vi "Main_maszyna.vi"() -> ()   [LabVIEW 2013]
doc: "Use this template to build a standard state machine design pattern. Each state executes code and determines which state to transition to. Contrast this design pattern with the User Interface Event Handler pattern, in which code executes in response to user actions. Contrast this design pattern also with the Queued Message Handler pattern, in which each message handling code can queue zero or more new messages.\nNote: This template does not contain the most recent programming guidelines recommended by National Instruments. For a complete, project-based implementation of the Standard State Machine pattern, use the Create Project dialog box instead of this template."
uses:
  inne pliki/Stany.ctl
  inne pliki/Params.ctl
  inne pliki/Data.ctl
  inne pliki/Akcje czas FVG.ctl
  <vilib>/Utility/error.llb/DialogType.ctl
  <vilib>/Utility/file.llb/Write To Spreadsheet File (DBL).vi
panel:
  out "path out":path
  in  "Generuj (F)":bool
  in  "Error?":bool
  out "Czas do końca pomiaru":dbl
  in  "bStopPomiar":bool
  out "Warning text":string
  out "Warning":bool
  in  "Temp limits":T1={"Max (25)"=22.0, "Min (0)"=0.0}
  out "Waveform Chart":cluster{"Temperatura":dbl, "Średnia":dbl}(graph)
  in  "Akcje":T2
  out "Stan aktualny":T3
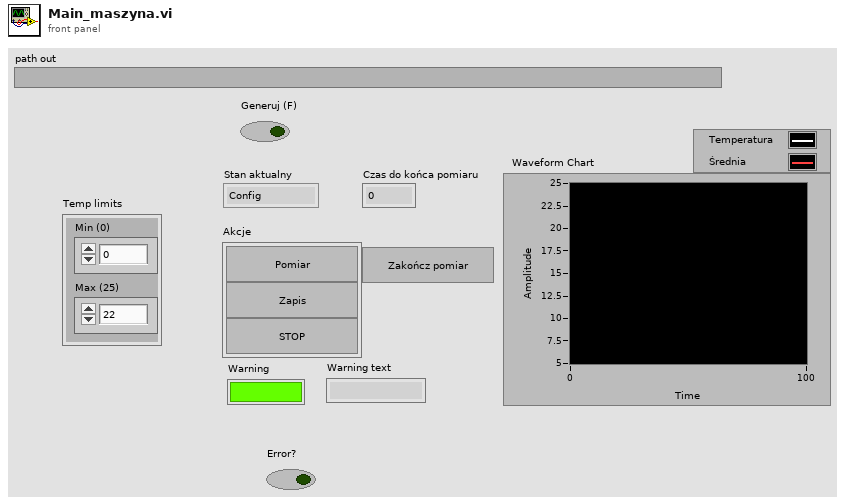
[diagram p1: front panel]
types:
  T1 = typedef "Params.ctl" = cluster{"Max (25)":dbl, "Min (0)":dbl}
  T2 = cluster{"bPomiar":bool, "bZapis":bool, "bSTOP":bool}
  T3 = typedef "Stany.ctl" = enum16{"Config", "IDLE", "Measure", "Analyze", "Display", "STOP", "Save", "Error", "Error end"}
  T4 = typedef "Data.ctl" = cluster{"Temperatura":dbl, "Średnia":dbl, "Warning":bool, "Warning text ":string, "Temp limits":T1, "Temp Array":dbl[], "Sternia Array":dbl[]}
  T5 = typedef "Akcje czas FVG.ctl" = enum16{"Reset", "Wait"}
  T6 = typedef "DialogType.ctl" = u16
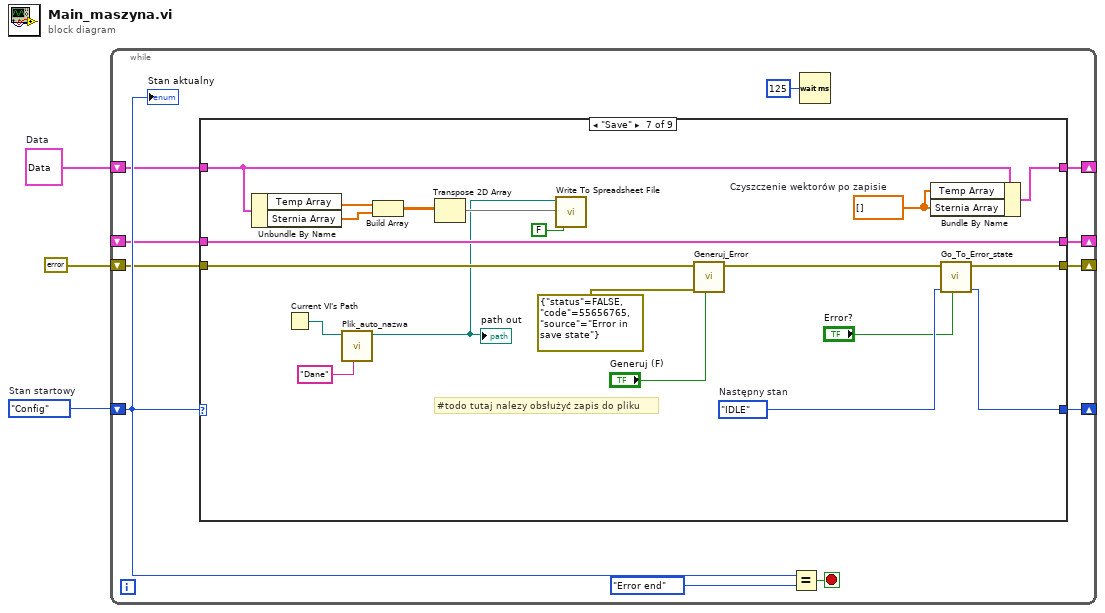
[diagram p0: block diagram]
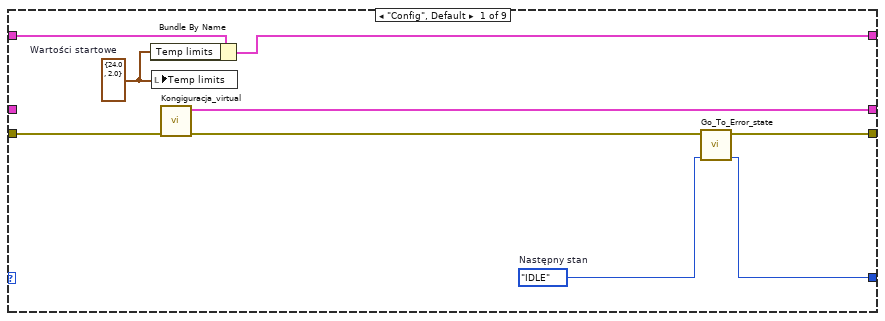
[diagram p2: hidden frame]
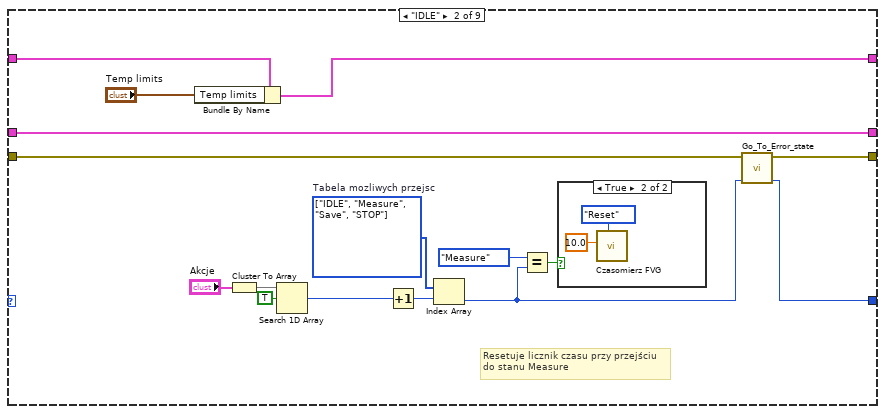
[diagram p3: hidden frame]
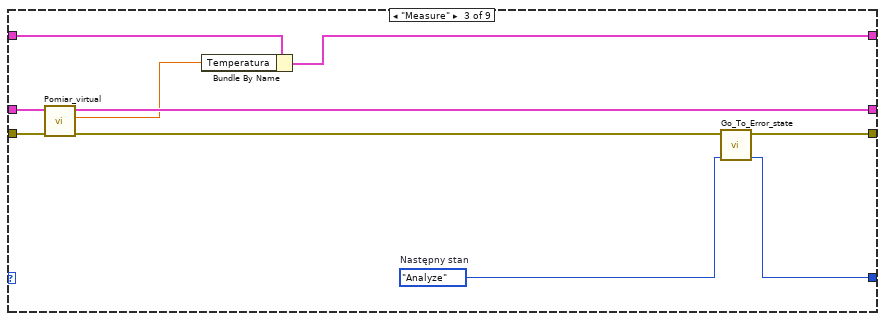
[diagram p5: hidden frame]
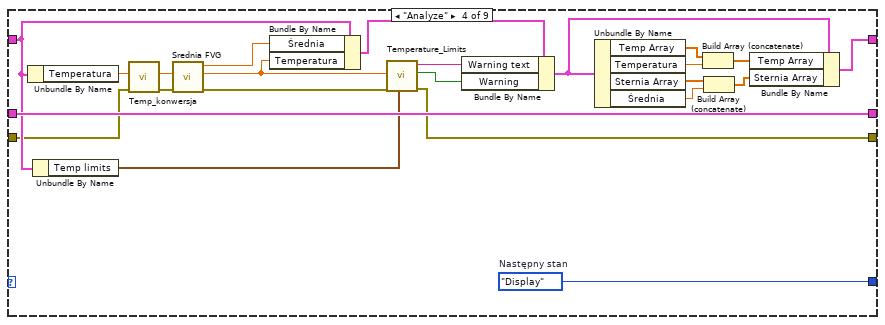
[diagram p6: hidden frame]
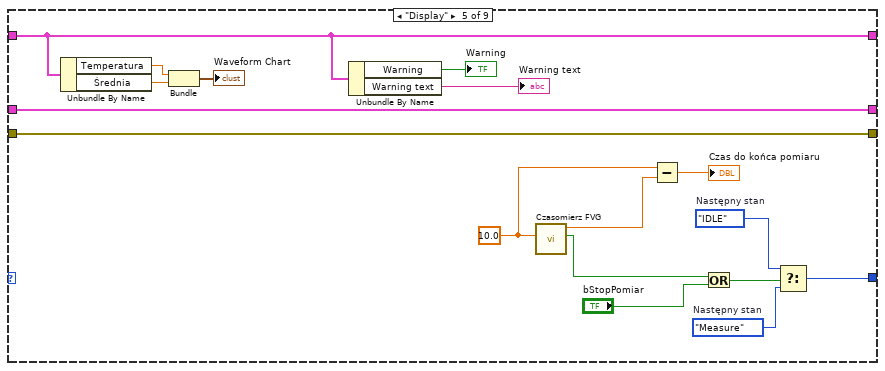
[diagram p7: hidden frame]
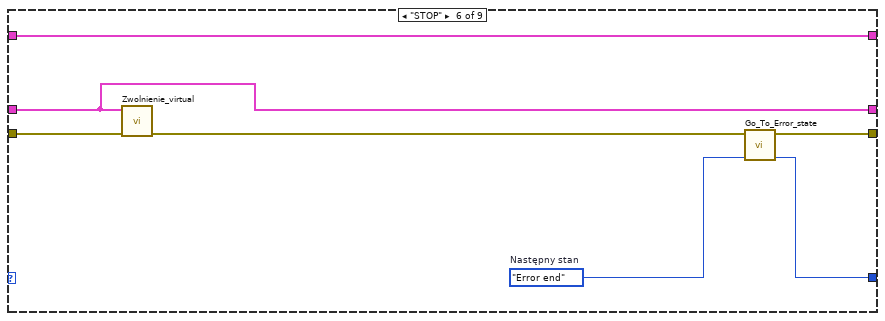
[diagram p8: hidden frame]
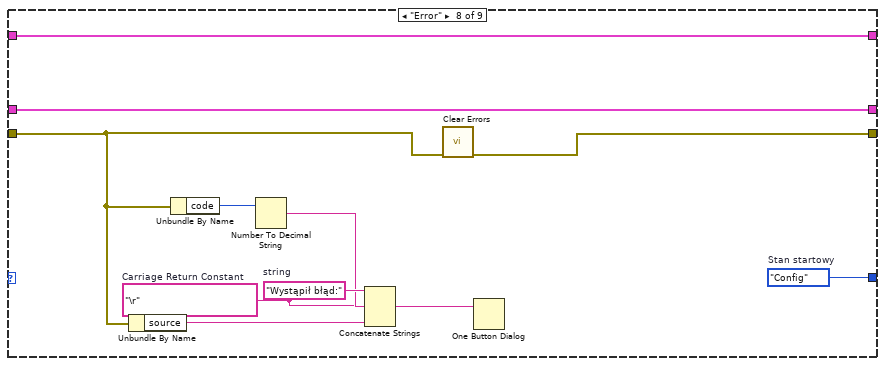
[diagram p9: hidden frame]
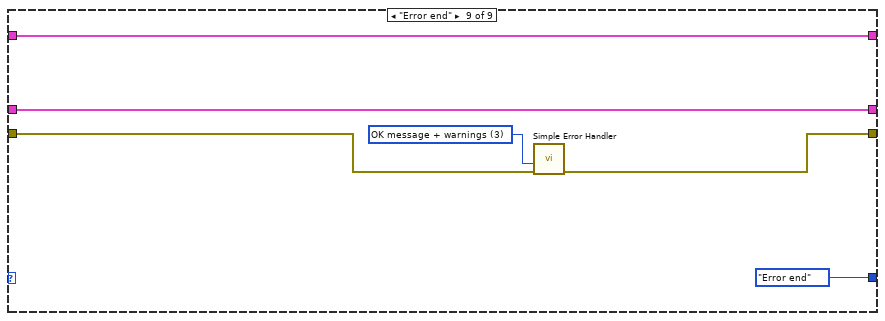
[diagram p10: hidden frame]
diagram:
  w2 = T4 {"Temperatura"=0.0, "Średnia"=0.0, "Warning"=FALSE, "Warning text "="", "Temp limits"={"Max (25)"=25.0, "Min (0)"=0.0}, "Temp Array"=[], "Sternia Array"=[]}  # Data
  w3 = Stany."Config"  # Stan startowy
  n1 = while {
    shift-right: [w12] -> _
    shift-left: w3 -> [w13]
    shift-right: [w8] -> _
    shift-left: w2 -> [w9]
    shift-right: [w7] -> _
    shift-left: _ -> [w6]
    shift-right: [w5] -> _
    shift-left: errorcluster {"status"=FALSE, "code"=0, "source"=""} ("error out") -> [w4]
    stop <- w14 stop-if-true
    n2 = case shown="\"Save\"" w13 {
      tunnel: [w16 w24 w42 w74 w82 w92 w114 w126 Stany."Error end" ("Stan startowy")] -> w12
      tunnel: w9 -> [w21 w31 w47 w70 w86 w98 w108 w129 w135]
      tunnel: [w20 w30 w46 w52 w86 w98 w117 w129 w135] -> w8
      tunnel: [w23 w33 w50 w73 w91 w96 w118 w128 w134] -> w7
      tunnel: w6 -> [_ w33 w51 w73 w91 w96 w118 w128 w134]
      tunnel: [w17 w27 w45 w65 w90 w95 w115 w127 w131] -> w5
      tunnel: w4 -> [w22 w26 w49 w66 w90 w97 w102 w119 w132]
      frame "Config", Default {
        w19 = T1 {"Max (25)"=24.0, "Min (0)"=2.0}  # Wartości startowe
        w15 = Stany."IDLE"  # Następny stan
        n3 = Bundle By Name(cluster=w21, "Temp limits"=w19) -> (w20:T4)
        n4 = local write "Temp limits"(w19) -> ()
        n5 = call "Kongiguracja_virtual.vi"("error in (no error)"=w22) -> ("error out"=w18:errorcluster, "Reference out"=w23:cluster{"Numeric":dbl, "Boolean":bool})  [unwired: 9 in]
        n6 = call "Go_To_Error_state.vi"("Następny stan in"=w15, "error in (no error)"=w18) -> ("Następny stan out"=w16:T3, "error out"=w17:errorcluster)  [unwired: 8 in]
      }
      frame "IDLE" {
        w34 = T3[] [enum."IDLE", enum."Measure", enum."Save", enum."STOP"] items=["Config", "IDLE", "Measure", "Analyze", "Display", "STOP", "Save", "Error", "Error end"]  # Tabela mozliwych przejsc
        # "Resetuje licznik czasu przy przejściu\ndo stanu Measure"
        n7 = Bundle By Name(cluster=w31, "Temp limits"="Temp limits") -> (w30:T4)
        n8 = Cluster To Array(cluster="Akcje") -> (array=w38:bool[])
        n9 = Search 1D Array(1D array=w38, element=TRUE) -> (index of element=w36:i32)  [unwired: 1 in]
        n10 = Increment(x=w36) -> (x+1=w35:i32)
        n11 = Index Array(array=w34, index=w35) -> (element=w25:T3)
        n12 = Equal?(x=Stany."Measure" ("Następny stan"), y=w25) -> (x = y?=w29:bool)
        n13 = case shown="True" w29 {
          frame False {
          }
          frame True {
            n14 = call "Czasomierz FVG.vi"("Akcja (Wait)"=Akcje_czas_FVG."Reset", "Czas (s)"=10.0) -> ()  [unwired: 7 in, 3 out]
          }
        }
        n15 = call "Go_To_Error_state.vi"("Następny stan in"=w25, "error in (no error)"=w26) -> ("Następny stan out"=w24:T3, "error out"=w27:errorcluster)  [unwired: 8 in]
      }
      frame "Measure" {
        w43 = Stany."Analyze"  # Następny stan
        n16 = call "Pomiar_virtual.vi"("error in (no error)"=w49, "Reference in"=w51) -> ("error out"=w44:errorcluster, "out"=w48:dbl, "Reference out"=w50:cluster{"Numeric":dbl, "Boolean":bool})  [unwired: 7 in]
        n17 = Bundle By Name(cluster=w47, "Temperatura"=w48) -> (w46:T4)
        n18 = call "Go_To_Error_state.vi"("Następny stan in"=w43, "error in (no error)"=w44) -> ("Następny stan out"=w42:T3, "error out"=w45:errorcluster)  [unwired: 8 in]
      }
      frame "Analyze" {
        w74 = Stany."Display"  # Następny stan
        n19 = Unbundle By Name(w70) -> ("Temperatura"=w72:dbl)
        n20 = Unbundle By Name(w70) -> ("Temp limits"=w71:T1)
        n21 = call "Temp_konwersja.vi"("error in (no error)"=w66, "Temp in"=w72) -> ("error out"=w64:errorcluster, "Temp out"=w63:dbl)  [unwired: 8 in]
        n22 = call "Srednia FVG.vi"("error in (no error)"=w64, "temperatura in"=w63) -> ("error out"=w62:errorcluster, "temperatura out"=w61:dbl, "średnia out"=w60:dbl)  [unwired: 7 in]
        n23 = Bundle By Name(cluster=w70, "Średnia"=w60, "Temperatura"=w61) -> (w67:T4)
        n24 = call "Temperature_Limits.vi"("Temp limits"=w71, "error in (no error)"=w62, "TEMP"=w61) -> ("error out"=w65:errorcluster, "Warning"=w68:bool, "Warning Text"=w69:string)  [unwired: 6 in]
        n25 = Bundle By Name(cluster=w67, "Warning text"=w69, "Warning"=w68) -> (w53:T4)
        n26 = Unbundle By Name(w53) -> ("Temp Array"=w59:dbl[], "Temperatura"=w58:dbl, "Sternia Array"=w57:dbl[], "Średnia"=w56:dbl)
        n27 = Build Array (concatenate)(w59, w58) -> (w55:dbl[])
        n28 = Build Array (concatenate)(w57, w56) -> (w54:dbl[])
        n29 = Bundle By Name(cluster=w53, "Temp Array"=w55, "Sternia Array"=w54) -> (w52:T4)
      }
      frame "Display" {
        w77 = 10.0 ("Czas (s)")
        w81 = Stany."Measure"  # Następny stan
        w83 = Stany."IDLE"  # Następny stan
        n30 = Unbundle By Name(w86) -> ("Temperatura"=w88:dbl, "Średnia"=w89:dbl)
        n31 = Bundle("Temperatura"=w88, "Średnia"=w89) -> (→"Waveform Chart":cluster{"Temperatura":dbl, "Średnia":dbl})  [unwired: 1 in]
        n32 = Unbundle By Name(w86) -> ("Warning"=→"Warning":bool, "Warning text"=→"Warning text":string)
        n33 = call "Czasomierz FVG.vi"("Czas (s)"=w77) -> ("Elapsed?"=w78:bool, "Elapsed Time"=w76:dbl)  [unwired: 8 in, 1 out]
        n34 = Subtract(x=w77, y=w76) -> (x-y=→"Czas do końca pomiaru":dbl)
        n35 = Or(x=w78, y="bStopPomiar") -> (x .or. y?=w80:bool)
        n36 = Select(t=w83, s=w80, f=w81) -> (s? t:f=w82:T3)
      }
      frame "STOP" {
        w93 = Stany."Error end"  # Następny stan
        n37 = call "Zwolnienie_virtual.vi"("error in (no error)"=w97, "Reference in"=w96) -> ("error out"=w94:errorcluster)  [unwired: 9 in]
        n38 = call "Go_To_Error_state.vi"("Następny stan in"=w93, "error in (no error)"=w94) -> ("Następny stan out"=w92:T3, "error out"=w95:errorcluster)  [unwired: 8 in]
      }
      frame "Save" {
        w116 = dbl[] []  # Czyszczenie wektorów po zapisie
        w113 = Stany."IDLE"  # Następny stan
        # "#todo tutaj nalezy obsłużyć zapis do pliku"
        n39 = Unbundle By Name "Unbundle By Name"(w108) -> ("Temp Array"=w107:dbl[], "Sternia Array"=w106:dbl[])
        n40 = Current VI's Path() -> (path=w103:path)
        n41 = call "Plik_auto_nazwa.vi"("Nazwa in"="Dane", "path in"=w103) -> ("path out"=w100:path)  [unwired: 8 in, 1 out]
        "path out" <- w100
        n42 = Build Array "Build Array"(w107, w106) -> (w105:dbl[][])
        n43 = Transpose 2D Array(2D array=w105) -> (transposed array=w104:dbl[][])
        n44 = call-poly <vilib>:"Write To Spreadsheet File.vi"("append to file? (new file:F)"=FALSE, "2D data"=w104, "file path (dialog if empty)"=w100) -> ()  [unwired: 5 in, 1 out]
        n45 = call "Generuj_Error.vi"("Generuj (F)"="Generuj (F)", "Generator"=errorcluster {"status"=FALSE, "code"=55656765, "source"="Error in save state"}, "error in (no error)"=w102) -> ("error out"=w111:errorcluster)  [unwired: 8 in]
        n46 = Bundle By Name(cluster=w108, "Temp Array"=w116, "Sternia Array"=w116) -> (w117:T4)
        n47 = call "Go_To_Error_state.vi"("GoTo Error (F)"="Error?", "Następny stan in"=w113, "error in (no error)"=w111) -> ("Następny stan out"=w114:T3, "error out"=w115:errorcluster)  [unwired: 7 in]
      }
      frame "Error" {
        w122 = "\r"  # Carriage Return Constant
        w124 = "Wystąpił błąd:"  # string
        w126 = Stany."Config"  # Stan startowy
        n48 = Unbundle By Name(w119) -> ("source"=w120:string)
        n49 = Unbundle By Name(w119) -> ("code"=w125:i32)
        n50 = Number To Decimal String(number=w125) -> (decimal integer string=w123:string)  [unwired: 1 in]
        n51 = Concatenate Strings "Concatenate Strings"(w124, w122, w123, w122, w120) -> (w121:string)
        n52 = call <vilib>:"Clear Errors.vi"("error in (no error)"=w119) -> ("error out"=w127:errorcluster)  [unwired: 6 in]
        n53 = One Button Dialog(message=w121) -> ()  [unwired: 1 in, 1 out]
      }
      frame "Error end" {
        w130 = T6 3 items=["no dialog", "OK message", "continue or stop message", "OK message + warnings", "continue/stop + warnings"] ("type of dialog (OK msg:1)")
        n54 = call <vilib>:"Simple Error Handler.vi"("type of dialog (OK msg:1)"=w130, "error in (no error)"=w132) -> ("error out"=w131:errorcluster)  [unwired: 3 in, 4 out]
      }
    }
    n55 = Equal?(x=w13, y=Stany."Error end" ("Stan startowy")) -> (x = y?=w14:bool)
    n56 = Wait (ms)(milliseconds to wait=u32 125) -> ()  [unwired: 1 out]
    "Stan aktualny" <- w13
  }
